vi "Find Value from Key (JSON Numeric).vi"(8 "error in (no error)":errorcluster, 10 "key":string, 11 "JSON Object in":refnum<class "JSON Object.lvclass">) -> (0 "error out":errorcluster, 2 "value":refnum<class "JSON Numeric.lvclass">)   [LabVIEW 2015, in "LVJSON.lvlib" / "JSON Object.lvclass"]
uses:
  JSON Object.lvclass
  JSON Numeric/JSON Numeric.lvclass
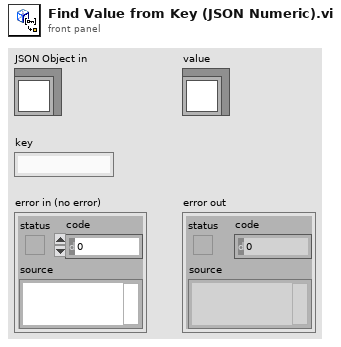
[diagram p1: front panel]
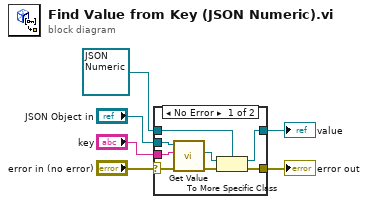
[diagram p0: block diagram]
diagram:
  n1 = case shown="No Error" "error in (no error)" {
    selector: "error in (no error)" -> [w12 w16]
    tunnel: [w8 w16] -> w5
    tunnel: "JSON Object in" -> [w14 _]
    tunnel: "key" -> [w13 _]
    tunnel: [w10 w15] -> w1
    tunnel: refnum<class "JSON Numeric.lvclass"> refnum ("JSON Numeric.lvclass") -> [w7 w15]
    frame No Error {
      n2 = call "Get Value.vi"("error in (no error)"=w12, "key"=w13, "JSON Object in"=w14) -> ("error out"=w9:errorcluster, "value"=w11:refnum<class "JSON Datatype.lvclass">)  [unwired: 7 in]
      n3 = To More Specific Class(target class=w7, reference=w11, error in=w9) -> (specific class reference=w10:refnum<class "JSON Numeric.lvclass">, error out=w8:errorcluster)
    }
    frame Error {
    }
  }
  "error out" <- w5
  "value" <- w1
